vi "configuration UI.vi"() -> ()   [LabVIEW 2014, in "io editor node.lvclass"]
uses:
  io editor node.lvclass
  <vilib>/NI/Module Execution Interface/Engine Configuration/engine configuration.lvclass
  <vilib>/NI/DCAF/Modules/UI/configuration/UI Reference configuration.lvclass
  <vilib>/NI/Configuration Framework/Controls/EventCluster.ctl
  <vilib>/NI/Configuration Framework/NISE_CEF_TreeControl.lvlib
  <vilib>/NI/Tag Bus/tag/tag descriptor.lvclass
  <vilib>/NI/Tag Bus/tag/Data Type.ctl
  <vilib>/NI/DCAF/Tag Editor Core/Configuration Editor/Classes/Module editor node/module editor node.lvclass
  <vilib>/NI/DCAF/Tag Editor Core/Configuration Editor/Classes/Engine Parent/Engine Parent Editor Node.lvclass
  configuration/io configuration.lvclass
  <vilib>/NI/Tools/Keyed Array/KeyedArray.ctl
  <vilib>/NI/Tools/Keyed Array/Tools_KeyedArray.lvlib
  <vilib>/NI/AMC/Message.ctl
  <vilib>/NI/AMC/AMC.lvlib
  <vilib>/NI/AMC/Message Queue.ctl
  <vilib>/NI/Configuration Framework/Node/NISE_CEF_Node.lvclass
  <vilib>/NI/Configuration Framework/Node/NodeRef.ctl
  <vilib>/NI/Configuration Framework/Node/UserEventRef.ctl
panel:
  in  "Gen from VI":bool
  in  "Browse VI":bool
  out "VI":string
  in  "Tab Control":enum32{"Static Configuration"}(tab)
  in  "Bitfile exe dir":path caption="Directory"
  in  "Load FPGA":bool=TRUE
  in  "Resource":string
  in  "Gen from Bitfile":bool
  in  "Browse Bitfile":bool
  out "Bitfile":string
  in  "hidden_remove":bool
  in  "hidden_settings":bool
  in  "hidden_Add":bool
  in  "Remove Button":bool
  in  "Add Button":bool
  in  "channel":i32(listbox)
  in  "settings":bool
  in  "user event":T1
  in  "main queue":T2
  in  "node ref":T3
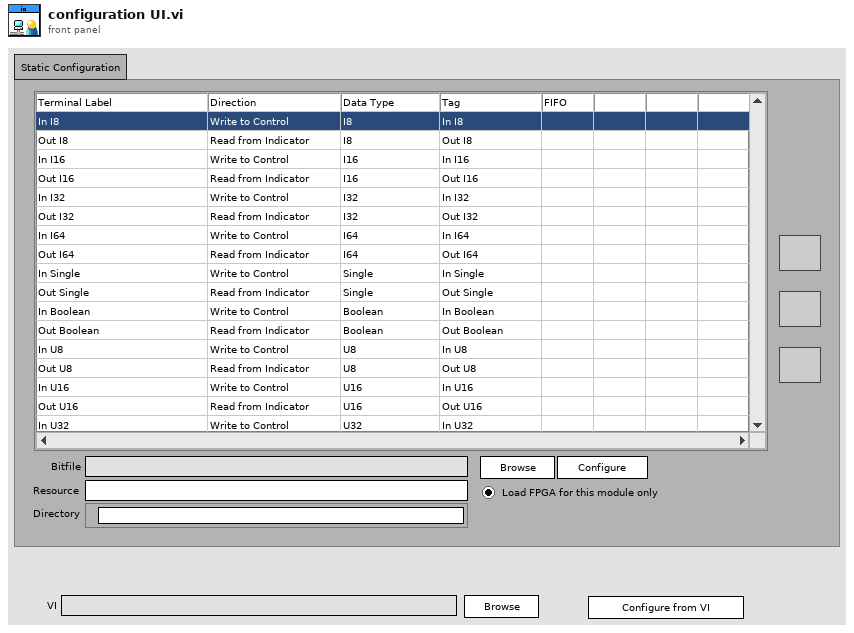
[diagram p1: front panel]
types:
  T1 = typedef "NISE_CEF_Node.lvclass/UserEventRef.ctl" = refnum<user-event>
  T2 = typedef "AMC.lvlib/Message Queue.ctl" = refnum<queue>
  T3 = typedef "NISE_CEF_Node.lvclass/NodeRef.ctl" = refnum<data-value>
  T4 = typedef "NISE_CEF_TreeControl.lvlib/EventCluster.ctl" = cluster{"command":string, "data":string}
  T5 = typedef "tag bus.lvlib/tag descriptor.lvclass/Data Type.ctl" = enum16{"Double", "Single", "I64", "I32", "I16", "I8", "U64", "U32", "U16", "U8", "Boolean", "String", "Array of Double", "Array of Single", "Array of I64", "Array of I32", "Array of I16", "Array of I8", "Array of U64", "Array of U32", "Array of U16", "Array of U8", "Array of Boolean", "Array of String"}
  T6 = typedef "io editor node.lvclass/table line.ctl" = cluster{"channel":refnum<class "TBM channel.lvclass">, "tag name":string}
  T7 = typedef "LVPoint32TypeDef.ctl" = cluster{"Horizontal":i32, "Vertical":i32}
  T8 = typedef "LVRowAndColumnTypeDef.ctl" = cluster{"Row":i32, "Column":i32}
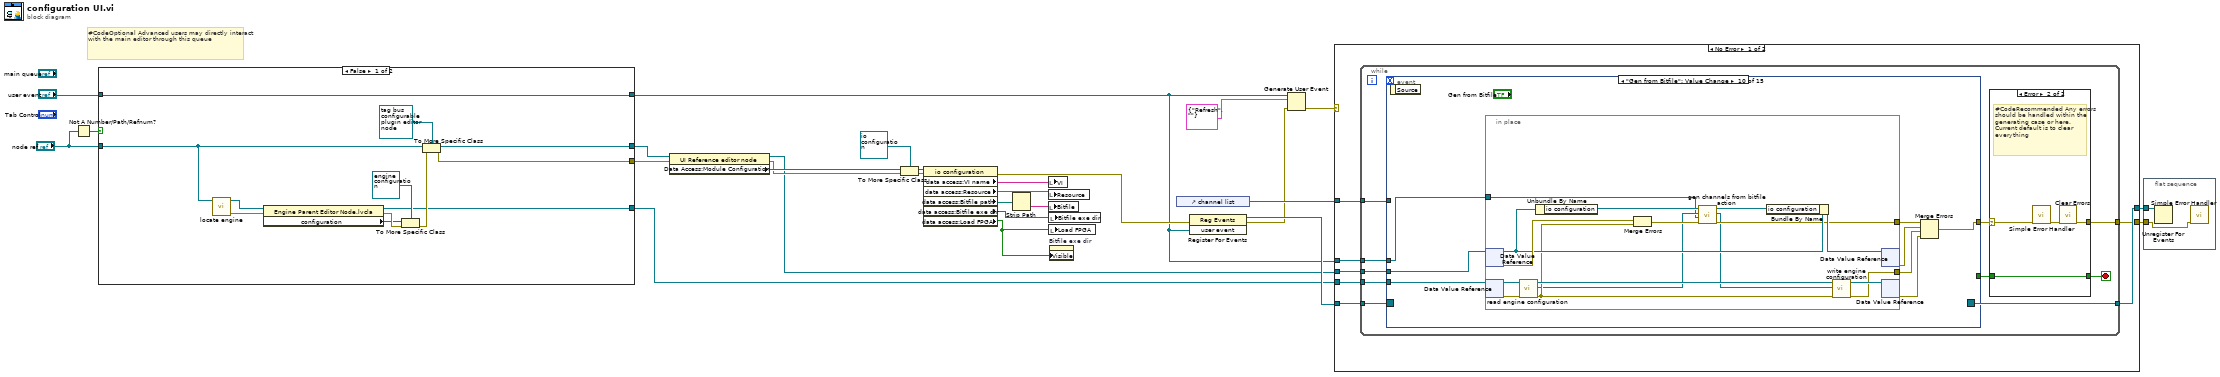
[diagram p0: block diagram]
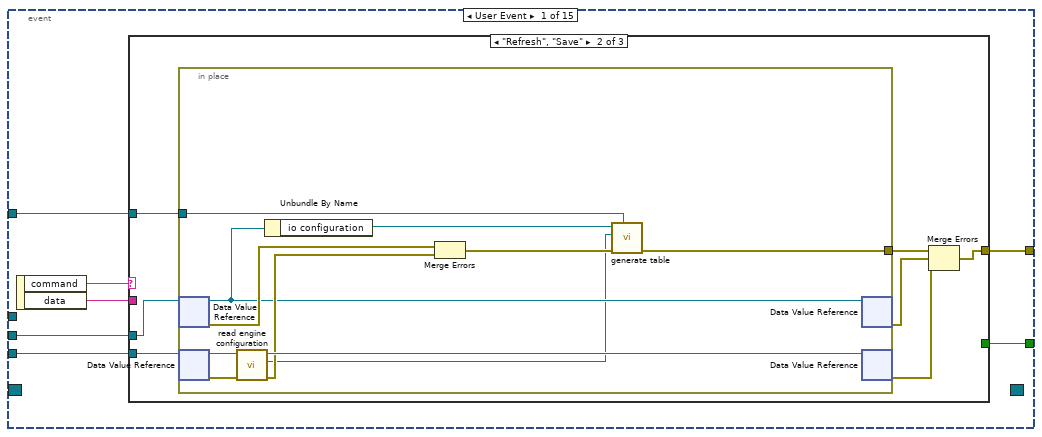
[diagram p3: hidden frame]
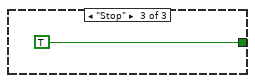
[diagram p5: hidden frame]
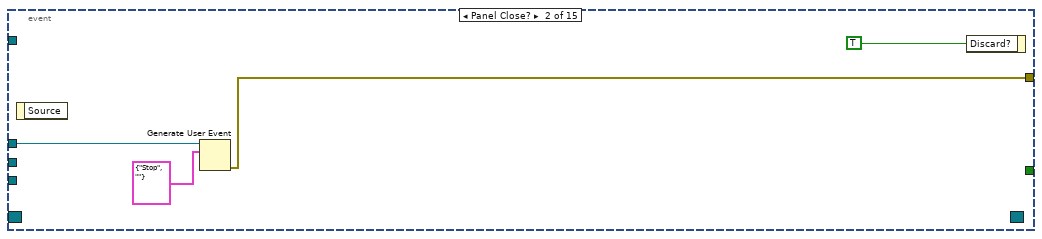
[diagram p6: hidden frame]
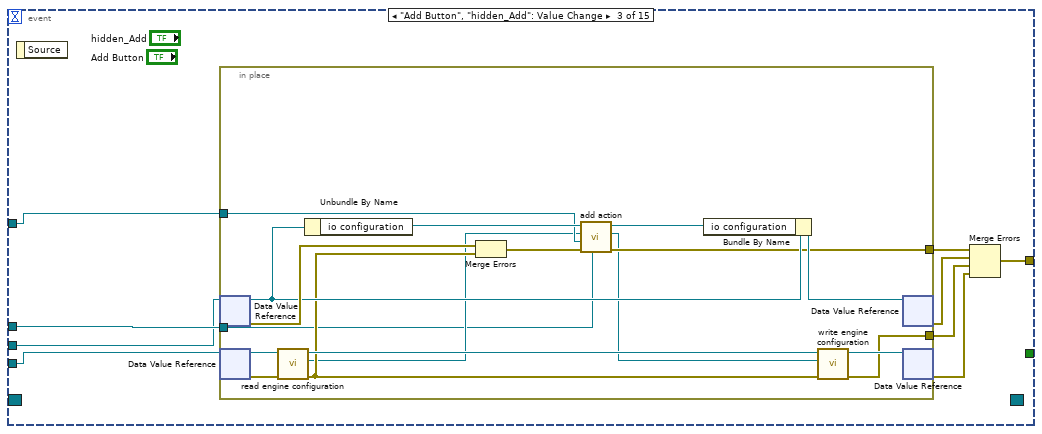
[diagram p7: hidden frame]
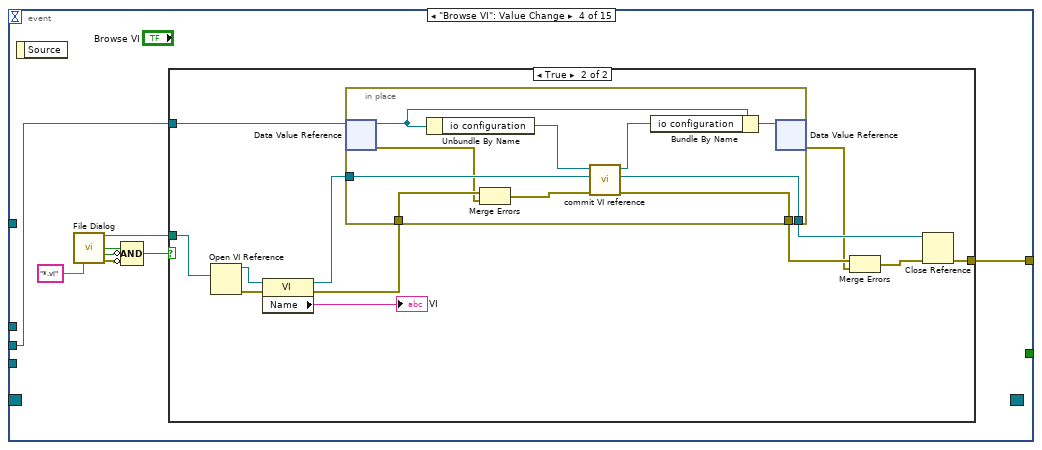
[diagram p8: hidden frame]
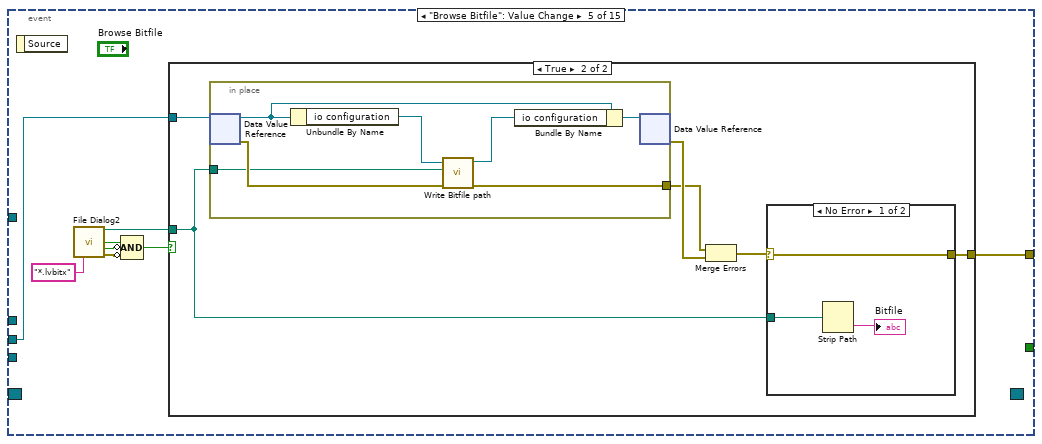
[diagram p10: hidden frame]
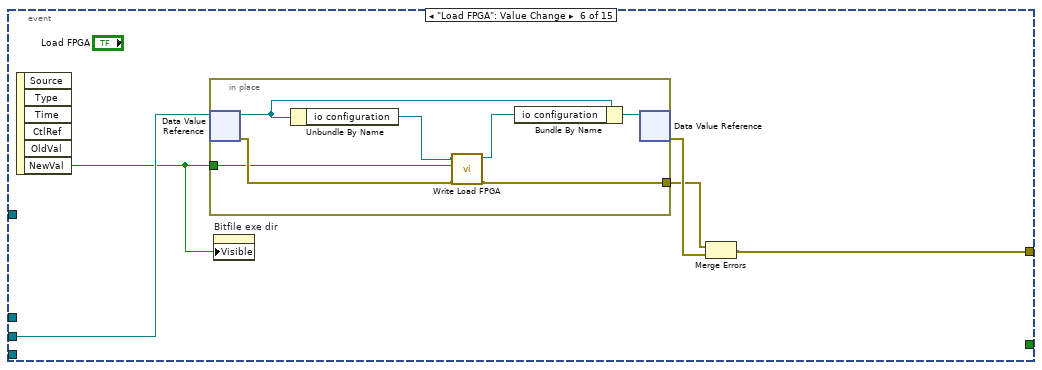
[diagram p13: hidden frame]
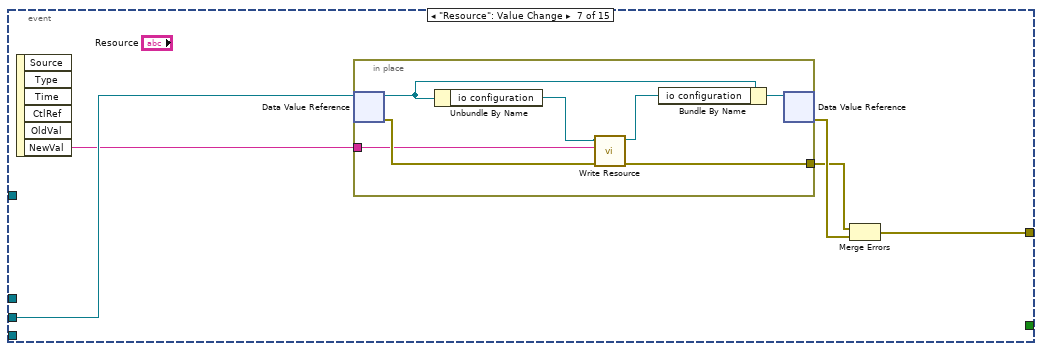
[diagram p14: hidden frame]
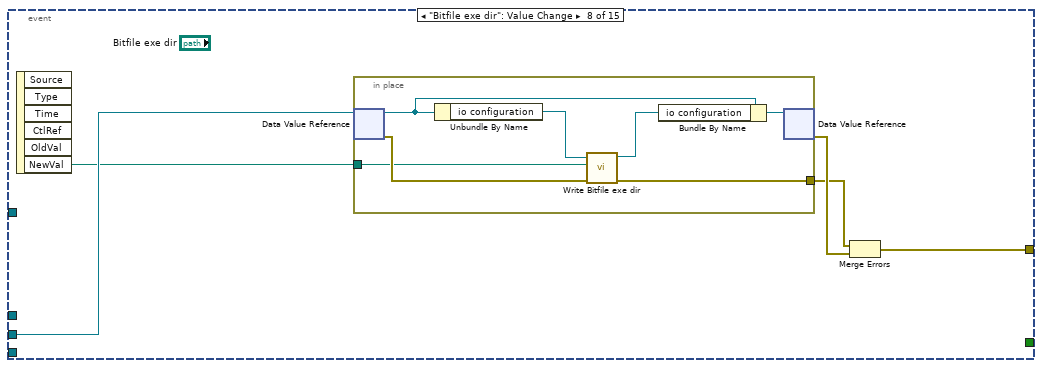
[diagram p15: hidden frame]
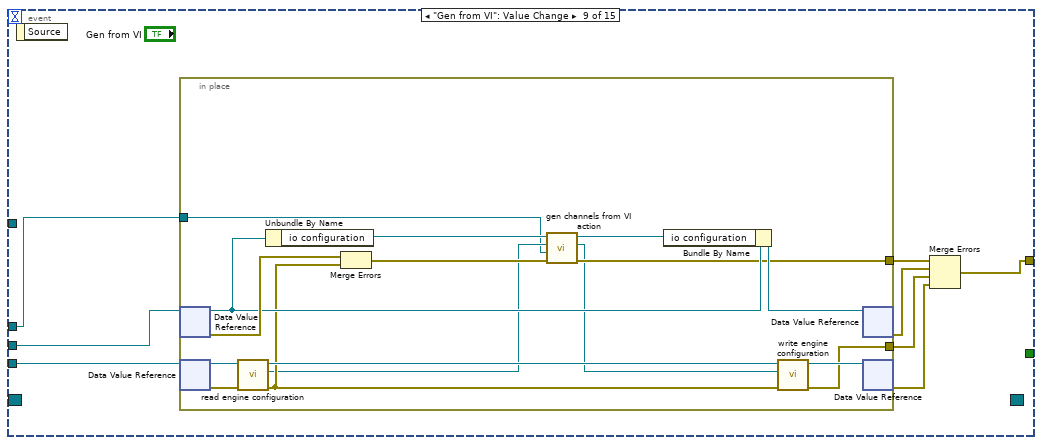
[diagram p16: hidden frame]
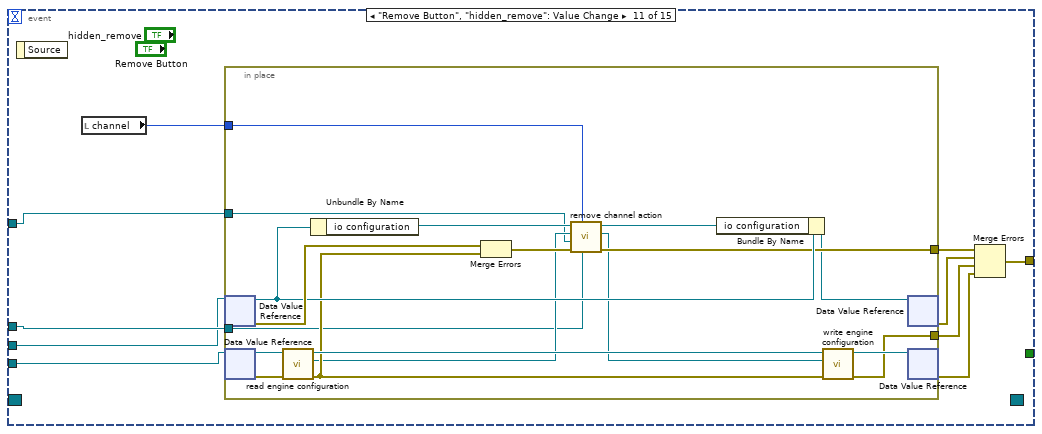
[diagram p17: hidden frame]
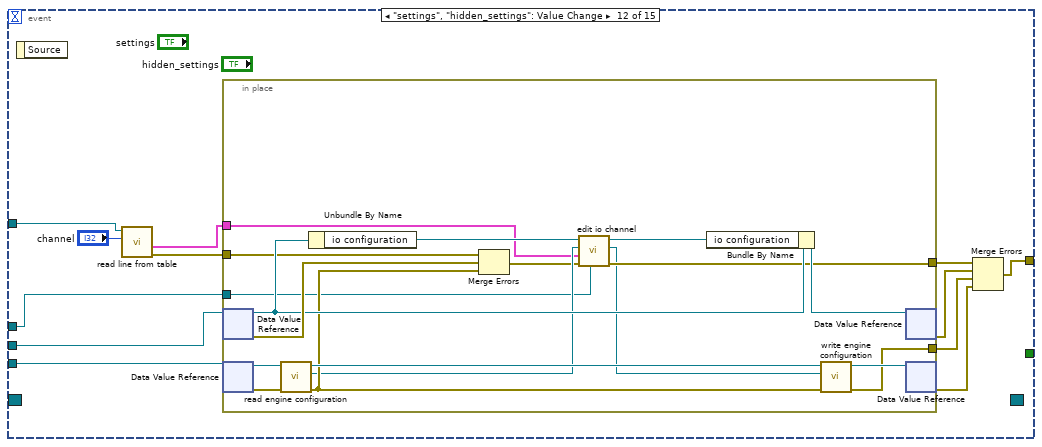
[diagram p18: hidden frame]
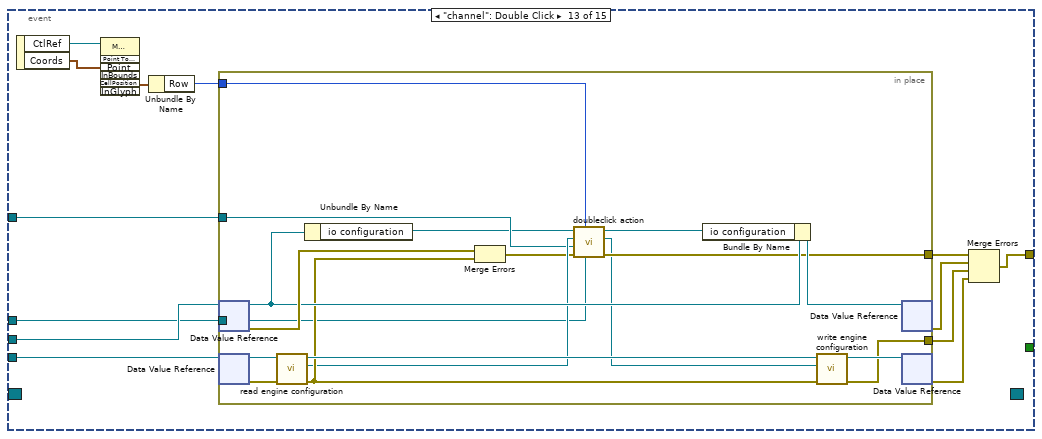
[diagram p19: hidden frame]
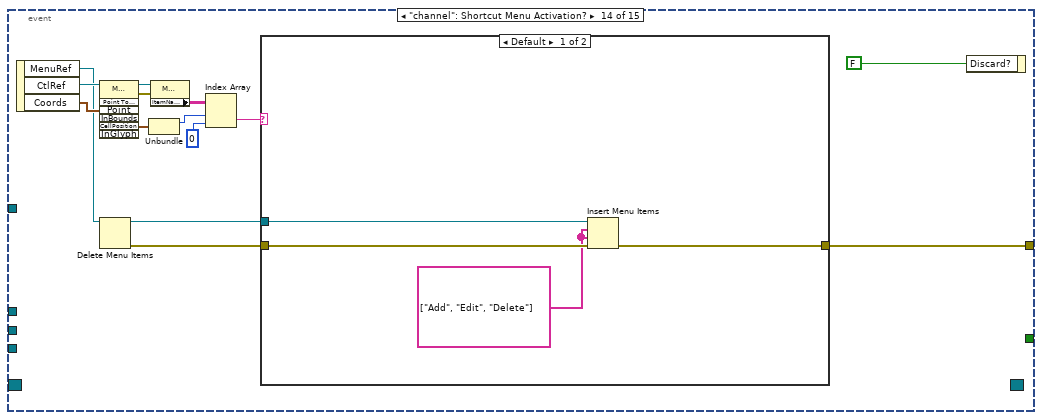
[diagram p20: hidden frame]
diagram:
  # "#CodeOptional Advanced users may directly interact with the main editor through this queue"
  n1 = Not A Number/Path/Refnum?(number/path/refnum="node ref") -> (NaN/Path/Refnum?=w21:bool)
  n2 = case shown="False" w21 {
    tunnel: "user event" -> [w39 w45]
    tunnel: [w39 w46] -> w9
    tunnel: "node ref" -> [w37 _]
    tunnel: [w36 w61] -> w16
    tunnel: [w35 w43] -> w19
    tunnel: [w28 w41] -> w14
    frame False {
      n3 = call <vilib>:"locate engine.vi"("component"=w37) -> ("error out"=w32:errorcluster, "engine"=w34:refnum<data-value>)  [unwired: 9 in]
      n4 = property class="Engine Parent Editor Node.lvcla"(reference=w34, error in=w32) -> (reference out=w28:refnum<data-value>, error out=w31:errorcluster, "configuration"=w30:refnum<class "NISE_CEF_serializable configuration.lvclass">)
      n5 = To More Specific Class(target class=refnum<class "engine configuration.lvclass"> refnum ("engine configuration.lvclass"), reference=w30, error in=w31) -> (error out=w29:errorcluster)  [unwired: 1 out]
      n6 = To More Specific Class(target class=refnum<data-value> refnum ("data value reference"), reference=w37, error in=w29) -> (specific class reference=w36:refnum<data-value>, error out=w35:errorcluster)
    }
    frame True {
      n7 = New Data Value Reference(data value=refnum<class "io editor node.lvclass"> refnum ("tag bus configurable plugin editor node")) -> (data value reference=w60:refnum<data-value>, error out=w63:errorcluster)  [unwired: 1 in]
      n8 = call-dynamic "Initialize.vi"("Engine in"=refnum<class "Engine Parent Editor Node.lvclass"> refnum) -> ("data value reference"=w59:T3)  [unwired: 8 in, 2 out]
      n9 = Create User Event(user event datatype=T4 {"command"="", "data"=""} ("event data"), error in=w63) -> (user event=w66:refnum<user-event>, error out=w62:errorcluster)
      n10 = property class="tag descriptor"(reference=refnum<class "tag descriptor.lvclass"> refnum ("tag descriptor"), "accessors:name"="mydouble" ("name"), "accessors:data type"=Data_Type."Double" ("data type")) -> (reference out=w47:refnum<class "tag descriptor.lvclass">)  [unwired: 1 in, 1 out]
      n11 = To More Specific Class(target class=refnum<data-value> refnum ("data value reference"), reference=w59) -> (specific class reference=w42:refnum<data-value>)  [unwired: 1 in, 1 out]
      n12 = property class="UI Reference editor node"(reference=w60, error in=w62, "configuration"=refnum<class "UI Reference configuration.lvclass"> refnum ("tag bus configurable plugin module configuration")) -> (reference out=w61:refnum<data-value>, error out=w53:errorcluster)
      n13 = property class="tag descriptor"(reference=w47, "accessors:name"="mydouble2" ("name")) -> (reference out=w48:refnum<class "tag descriptor.lvclass">)  [unwired: 1 in, 1 out]
      n14 = Type Cast(type=w45, x=w66) -> (*(type *) &x=w46:T1)
      n15 = call-dynamic "add tag.vi"("error in"=w53, "tag descriptor"=w47, "engine configuration in"=refnum<class "engine configuration.lvclass"> refnum ("Engine Configuration")) -> ("error out"=w51:errorcluster, "engine configuration out"=w50:refnum<class "engine configuration.lvclass">)  [unwired: 7 in]
      n16 = call-dynamic "add tag.vi"("error in"=w51, "tag descriptor"=w48, "engine configuration in"=w50) -> ("error out"=w49:errorcluster, "engine configuration out"=w40:refnum<class "engine configuration.lvclass">)  [unwired: 7 in]
      n17 = property class="Engine Parent Editor Node.lvcla"(reference=w42, error in=w49, "Data Access:Engine Configuration"=w40) -> (reference out=w41:refnum<data-value>, error out=w43:errorcluster)
    }
  }
  n18 = property class="UI Reference editor node"(reference=w16, error in=w19) -> (reference out=w15:refnum<data-value>, error out=w22:errorcluster, "Data Access:Module Configuration"=w23:refnum<class "TBM module configuration.lvclass">)
  n19 = To More Specific Class(target class=refnum<class "io configuration.lvclass"> refnum ("tag bus configurable plugin module configuration"), reference=w23, error in=w22) -> (specific class reference=w11:refnum<class "io configuration.lvclass">, error out=w17:errorcluster)
  n20 = property class="io configuration"(reference=w11, error in=w17) -> (error out=w12:errorcluster, "data access:VI name"=w10:string, "data access:Resource"=w4:string, "data access:Bitfile path"=w5:path, "data access:Bitfile exe dir"=w2:path, "data access:Load FPGA"=w1:bool)  [unwired: 1 out]
  n21 = Strip Path(path=w5) -> (name=w3:string)  [unwired: 1 out]
  n22 = local write "VI"(w10) -> ()
  n23 = local write "Resource"(w4) -> ()
  n24 = local write "Bitfile"(w3) -> ()
  n25 = local write "Bitfile exe dir"(w2) -> ()
  n26 = local write "Load FPGA"(w1) -> ()
  n27 = property on="Bitfile exe dir" class="Path"("Visible"=w1) -> ()  [unwired: 2 in, 2 out]
  n28 = control-ref of="channel list"() -> (w13:refnum<vi>)
  n29 = register-events(error in=w12, w9) -> (reference out=w27:refnum<event-registration>, error out=w7:errorcluster)  [unwired: 1 in]
  n30 = Generate User Event(user event=w9, event data cluster=T4 {"command"="Refresh", "data"=""} ("event data"), error in=w7) -> (error out=w6:errorcluster)  [unwired: 1 in, 1 out]
  n31 = case shown="No Error" w6 {
    selector: w6 -> [_ w414]
    tunnel: w27 -> [w74 w415]
    tunnel: [w73 w415] -> w26
    tunnel: [w72 w414] -> w25
    tunnel: w15 -> [w71 _]
    tunnel: w14 -> [w70 _]
    tunnel: w13 -> [w69 _]
    tunnel: w9 -> [w68 _]
    frame No Error {
      n32 = while {
        tunnel: w74 -> [w84]
        tunnel: [w83] -> w73
        tunnel: w71 -> [w79]
        tunnel: w70 -> [w78]
        tunnel: w68 -> [w77]
        tunnel: w69 -> [w75]
        tunnel: [w80] -> w72
        stop <- w82 stop-if-true
        n33 = event shown="[9] \"Gen from Bitfile\": Value Change" {
          selector: w84 -> [_ _ _ _ _ _ _ _ _ _ _ _ _ _ _]
          dyn-events: [_ _ _ _ _ _ _ _ _ _ _ _ _ _ _] -> w83
          timeout: _ -> [_ _ _ _ _ _ _ _ _ _ _ _ _ _ _]
          tunnel: [w97 _ _ _ _ _ _ _ _ _ _ _ _ _ _] -> w81
          tunnel: [w92 w117 w125 w148 w177 w203 w217 w229 w241 w265 w291 w319 w349 w375 w400] -> w76
          tunnel: w79 -> [w95 _ w121 w147 w178 w206 w218 w230 w239 w263 w286 w317 w347 _ _]
          tunnel: w78 -> [w94 _ w124 _ _ _ _ _ w240 w264 w287 w318 w348 _ _]
          tunnel: w77 -> [_ w118 w122 _ _ _ _ _ w238 w262 w289 w315 w346 _ _]
          tunnel: w75 -> [w91 _ w123 _ _ _ _ _ _ _ w288 w324 w345 _ _]
          event User Event {
            n34 = event-data() -> ("command"=w96:string, "data"=w93:string)  [unwired: 1 in]
            n35 = case shown="\"Refresh\", \"Save\"" w96 {
              tunnel: [_ _ TRUE] -> w97
              tunnel: w95 -> [_ w100 _]
              tunnel: w94 -> [_ w101 _]
              tunnel: w93 -> [_ _ _]
              tunnel: [_ w102 _] -> w92
              tunnel: w91 -> [_ w103 _]
              frame Default {
              }
              frame "Refresh", "Save" {
                n36 = in-place {
                  in-place-border: [w115] -> w104
                  in-place-border: w103 -> [w114]
                  n37 = in-place-dvr #1(w100) -> (w107:refnum<class "io editor node.lvclass">, w108:errorcluster)
                  n38 = in-place-dvr #2(w101) -> (w112:refnum<class "Engine Parent Editor Node.lvclass">, w111:errorcluster)
                  n39 = call <vilib>:"read engine configuration.vi"("error in"=w111, "Engine Parent Editor Node in"=w112) -> ("error out"=w109:errorcluster, "engine configuration"=w105:refnum<class "engine configuration.lvclass">, "Engine Parent Editor Node out"=w110:refnum<class "Engine Parent Editor Node.lvclass">)  [unwired: 7 in]
                  n40 = Unbundle By Name(w107) -> ("io configuration"=w106:refnum<class "io configuration.lvclass">)
                  n41 = Merge Errors(w108, w109) -> (w113:errorcluster)
                  n42 = call "generate table.vi"("table"=w114, "error in"=w113, "engine configuration"=w105, "tag bus configurable plugin module configuration"=w106) -> ("error out"=w115:errorcluster)  [unwired: 7 in]
                  n43 = in-place-dvr #1(w107) -> (w98:errorcluster)  [unwired: 1 out]
                  n44 = in-place-dvr #2(w110) -> (w99:errorcluster)  [unwired: 1 out]
                }
                n45 = Merge Errors(w104, w98, w99) -> (w102:errorcluster)
              }
              frame "Stop" {
              }
            }
          }
          event Panel Close? {
            n46 = event-data() -> ()  [unwired: 1 in, 1 out]
            n47 = Generate User Event(user event=w118, event data cluster=T4 {"command"="Stop", "data"=""} ("event data")) -> (error out=w117:errorcluster)  [unwired: 2 in, 1 out]
            n48 = event-data("Discard?"=TRUE) -> ()  [unwired: 1 in, 1 out]
          }
          event "Add Button", "hidden_Add": Value Change {
            n49 = event-data() -> ()  [unwired: 1 in, 1 out]
            n50 = in-place {
              in-place-border: [w137] -> w126
              in-place-border: [w140] -> w129
              in-place-border: w123 -> [w132]
              in-place-border: w122 -> [w130]
              n51 = in-place-dvr #3(w121) -> (w143:refnum<class "io editor node.lvclass">, w144:errorcluster)
              n52 = in-place-dvr #4(w124) -> (w146:refnum<class "Engine Parent Editor Node.lvclass">, w145:errorcluster)
              n53 = call <vilib>:"read engine configuration.vi"("error in"=w145, "Engine Parent Editor Node in"=w146) -> ("error out"=w139:errorcluster, "engine configuration"=w131:refnum<class "engine configuration.lvclass">, "Engine Parent Editor Node out"=w142:refnum<class "Engine Parent Editor Node.lvclass">)  [unwired: 7 in]
              n54 = Unbundle By Name(w143) -> ("io configuration"=w133:refnum<class "io configuration.lvclass">)
              n55 = Merge Errors(w144, w139) -> (w136:errorcluster)
              n56 = call "add action.vi"("user event"=w130, "error in"=w136, "channel list"=w132, "engine configuration in"=w131, "io configuration in"=w133) -> ("error out"=w137:errorcluster, "engine configuration out"=w134:refnum<class "engine configuration.lvclass">, "io configuration out"=w135:refnum<class "io configuration.lvclass">)  [unwired: 4 in]
              n57 = Bundle By Name(cluster=w143, "io configuration"=w135) -> (w138:refnum<class "io editor node.lvclass">)
              n58 = call <vilib>:"write engine configuration.vi"("error in"=w139, "engine configuration"=w134, "Engine Parent Editor Node in"=w142) -> ("error out"=w140:errorcluster, "Engine Parent Editor Node out"=w141:refnum<class "Engine Parent Editor Node.lvclass">)  [unwired: 7 in]
              n59 = in-place-dvr #3(w138) -> (w128:errorcluster)  [unwired: 1 out]
              n60 = in-place-dvr #4(w141) -> (w127:errorcluster)  [unwired: 1 out]
            }
            n61 = Merge Errors(w126, w128, w129, w127) -> (w125:errorcluster)
          }
          event "Browse VI": Value Change {
            n62 = event-data() -> ()  [unwired: 1 in, 1 out]
            n63 = call "File Dialog"("pattern (all files)"="*.vi") -> ("selected path"=w149:path, "exists"=w153:bool, "cancelled"=w152:bool, "error out"=w151:errorcluster)  [unwired: 11 in]
            n64 = Compound Arithmetic op=AND(w153, invert w152, invert w151) -> (w150:bool)
            n65 = case shown="True" w150 {
              tunnel: w149 -> [_ w166]
              tunnel: [_ w162] -> w148
              tunnel: w147 -> [_ w157]
              frame False {
              }
              frame True {
                n66 = Open VI Reference(vi path=w166) -> (vi reference=w164:refnum<vi>, error out=w165:errorcluster)  [unwired: 5 in]
                n67 = property class="VI"(reference=w164, error in=w165) -> (reference out=w159:refnum<vi>, error out=w160:errorcluster, "Name"=→"VI":string)
                n68 = in-place {
                  in-place-border: [w176] -> w161
                  in-place-border: w160 -> [w175]
                  in-place-border: w159 -> [w174]
                  in-place-border: [w173] -> w158
                  n69 = in-place-dvr #5(w157) -> (w170:refnum<class "io editor node.lvclass">, w167:errorcluster)
                  n70 = Unbundle By Name(w170) -> ("io configuration"=w172:refnum<class "io configuration.lvclass">)
                  n71 = Merge Errors(w175, w167) -> (w168:errorcluster)
                  n72 = call "commit VI reference.vi"("error in"=w168, "VI Refnum in"=w174, "io configuration in"=w172) -> ("error out"=w173:errorcluster, "VI Refnum out"=w176:refnum<vi>, "io configuration out"=w169:refnum<class "io configuration.lvclass">)  [unwired: 6 in]
                  n73 = Bundle By Name(cluster=w170, "io configuration"=w169) -> (w171:refnum<class "io editor node.lvclass">)
                  n74 = in-place-dvr #5(w171) -> (w155:errorcluster)  [unwired: 1 out]
                }
                n75 = Merge Errors(w158, w155) -> (w156:errorcluster)
                n76 = Close Reference(reference=w161, error in (no error)=w156) -> (error out=w162:errorcluster)
              }
            }
          }
          event "Browse Bitfile": Value Change {
            n77 = event-data() -> ()  [unwired: 1 in, 1 out]
            n78 = call "File Dialog2"("pattern (all files)"="*.lvbitx") -> ("selected path"=w179:path, "exists"=w183:bool, "cancelled"=w182:bool, "error out"=w181:errorcluster)  [unwired: 11 in]
            n79 = Compound Arithmetic op=AND(w183, invert w182, invert w181) -> (w180:bool)
            n80 = case shown="True" w180 {
              tunnel: w179 -> [_ w186]
              tunnel: w178 -> [_ w190]
              tunnel: [_ w185] -> w177
              frame False {
              }
              frame True {
                n81 = in-place {
                  in-place-border: [w196] -> w188
                  in-place-border: w186 -> [w195]
                  n82 = in-place-dvr #6(w190) -> (w200:refnum<class "io editor node.lvclass">, w197:errorcluster)
                  n83 = Unbundle By Name(w200) -> ("io configuration"=w199:refnum<class "io configuration.lvclass">)
                  n84 = call "Write Bitfile path.vi"("error in (no error)"=w197, "Bitfile path"=w195, "io configuration in"=w199) -> ("error out"=w196:errorcluster, "io configuration out"=w198:refnum<class "io configuration.lvclass">)  [unwired: 7 in]
                  n85 = Bundle By Name(cluster=w200, "io configuration"=w198) -> (w201:refnum<class "io editor node.lvclass">)
                  n86 = in-place-dvr #6(w201) -> (w189:errorcluster)  [unwired: 1 out]
                }
                n87 = Merge Errors(w188, w189) -> (w187:errorcluster)
                n88 = case shown="No Error" w187 {
                  selector: w187 -> [w191 w194]
                  tunnel: w186 -> [w192 _]
                  tunnel: [w191 w194] -> w185
                  frame No Error {
                    n89 = Strip Path(path=w192) -> (name=→"Bitfile":string)  [unwired: 1 out]
                  }
                  frame Error {
                  }
                }
              }
            }
          }
          event "Load FPGA": Value Change {
            n90 = event-data() -> ("NewVal"=w202:bool)  [unwired: 1 in, 5 out]
            n91 = in-place {
              in-place-border: [w208] -> w204
              in-place-border: w202 -> [w207]
              n92 = in-place-dvr #7(w206) -> (w212:refnum<class "io editor node.lvclass">, w209:errorcluster)
              n93 = Unbundle By Name(w212) -> ("io configuration"=w211:refnum<class "io configuration.lvclass">)
              n94 = call "Write Load FPGA.vi"("error in (no error)"=w209, "Load FPGA"=w207, "io configuration in"=w211) -> ("error out"=w208:errorcluster, "io configuration out"=w210:refnum<class "io configuration.lvclass">)  [unwired: 7 in]
              n95 = Bundle By Name(cluster=w212, "io configuration"=w210) -> (w213:refnum<class "io editor node.lvclass">)
              n96 = in-place-dvr #7(w213) -> (w205:errorcluster)  [unwired: 1 out]
            }
            n97 = property on="Bitfile exe dir" class="Path"("Visible"=w202) -> ()  [unwired: 2 in, 2 out]
            n98 = Merge Errors(w204, w205) -> (w203:errorcluster)
          }
          event "Resource": Value Change {
            n99 = event-data() -> ("NewVal"=w214:string)  [unwired: 1 in, 5 out]
            n100 = in-place {
              in-place-border: [w220] -> w215
              in-place-border: w214 -> [w219]
              n101 = in-place-dvr #8(w218) -> (w224:refnum<class "io editor node.lvclass">, w221:errorcluster)
              n102 = Unbundle By Name(w224) -> ("io configuration"=w223:refnum<class "io configuration.lvclass">)
              n103 = call "Write Resource.vi"("error in (no error)"=w221, "Resource"=w219, "io configuration in"=w223) -> ("error out"=w220:errorcluster, "io configuration out"=w222:refnum<class "io configuration.lvclass">)  [unwired: 7 in]
              n104 = Bundle By Name(cluster=w224, "io configuration"=w222) -> (w225:refnum<class "io editor node.lvclass">)
              n105 = in-place-dvr #8(w225) -> (w216:errorcluster)  [unwired: 1 out]
            }
            n106 = Merge Errors(w215, w216) -> (w217:errorcluster)
          }
          event "Bitfile exe dir": Value Change {
            n107 = event-data() -> ("NewVal"=w226:path)  [unwired: 1 in, 5 out]
            n108 = in-place {
              in-place-border: [w232] -> w227
              in-place-border: w226 -> [w231]
              n109 = in-place-dvr #9(w230) -> (w236:refnum<class "io editor node.lvclass">, w233:errorcluster)
              n110 = Unbundle By Name(w236) -> ("io configuration"=w235:refnum<class "io configuration.lvclass">)
              n111 = call "Write Bitfile exe dir.vi"("error in (no error)"=w233, "Bitfile exe dir"=w231, "io configuration in"=w235) -> ("error out"=w232:errorcluster, "io configuration out"=w234:refnum<class "io configuration.lvclass">)  [unwired: 7 in]
              n112 = Bundle By Name(cluster=w236, "io configuration"=w234) -> (w237:refnum<class "io editor node.lvclass">)
              n113 = in-place-dvr #9(w237) -> (w228:errorcluster)  [unwired: 1 out]
            }
            n114 = Merge Errors(w227, w228) -> (w229:errorcluster)
          }
          event "Gen from VI": Value Change {
            n115 = event-data() -> ()  [unwired: 1 in, 1 out]
            n116 = in-place {
              in-place-border: [w252] -> w242
              in-place-border: [w255] -> w245
              in-place-border: w238 -> [w246]
              n117 = in-place-dvr #10(w239) -> (w258:refnum<class "io editor node.lvclass">, w259:errorcluster)
              n118 = in-place-dvr #11(w240) -> (w261:refnum<class "Engine Parent Editor Node.lvclass">, w260:errorcluster)
              n119 = call <vilib>:"read engine configuration.vi"("error in"=w260, "Engine Parent Editor Node in"=w261) -> ("error out"=w254:errorcluster, "engine configuration"=w250:refnum<class "engine configuration.lvclass">, "Engine Parent Editor Node out"=w257:refnum<class "Engine Parent Editor Node.lvclass">)  [unwired: 7 in]
              n120 = Unbundle By Name(w258) -> ("io configuration"=w249:refnum<class "io configuration.lvclass">)
              n121 = Merge Errors(w259, w254) -> (w251:errorcluster)
              n122 = call "gen channels from VI action.vi"("error in"=w251, "user event"=w246, "engine configuration in"=w250, "io configuration in"=w249) -> ("error out"=w252:errorcluster, "engine configuration out"=w247:refnum<class "engine configuration.lvclass">, "io configuration out"=w248:refnum<class "io configuration.lvclass">)  [unwired: 5 in]
              n123 = Bundle By Name(cluster=w258, "io configuration"=w248) -> (w253:refnum<class "io editor node.lvclass">)
              n124 = call <vilib>:"write engine configuration.vi"("error in"=w254, "engine configuration"=w247, "Engine Parent Editor Node in"=w257) -> ("error out"=w255:errorcluster, "Engine Parent Editor Node out"=w256:refnum<class "Engine Parent Editor Node.lvclass">)  [unwired: 7 in]
              n125 = in-place-dvr #10(w253) -> (w244:errorcluster)  [unwired: 1 out]
              n126 = in-place-dvr #11(w256) -> (w243:errorcluster)  [unwired: 1 out]
            }
            n127 = Merge Errors(w242, w244, w245, w243) -> (w241:errorcluster)
          }
          event "Gen from Bitfile": Value Change {
            n128 = event-data() -> ()  [unwired: 1 in, 1 out]
            n129 = in-place {
              in-place-border: [w276] -> w266
              in-place-border: [w279] -> w269
              in-place-border: w262 -> [w270]
              n130 = in-place-dvr #12(w263) -> (w282:refnum<class "io editor node.lvclass">, w283:errorcluster)
              n131 = in-place-dvr #13(w264) -> (w285:refnum<class "Engine Parent Editor Node.lvclass">, w284:errorcluster)
              n132 = call <vilib>:"read engine configuration.vi"("error in"=w284, "Engine Parent Editor Node in"=w285) -> ("error out"=w278:errorcluster, "engine configuration"=w274:refnum<class "engine configuration.lvclass">, "Engine Parent Editor Node out"=w281:refnum<class "Engine Parent Editor Node.lvclass">)  [unwired: 7 in]
              n133 = Unbundle By Name(w282) -> ("io configuration"=w273:refnum<class "io configuration.lvclass">)
              n134 = Merge Errors(w283, w278) -> (w275:errorcluster)
              n135 = call "gen channels from bitfile action.vi"("error in"=w275, "user event"=w270, "engine configuration in"=w274, "io configuration in"=w273) -> ("error out"=w276:errorcluster, "engine configuration out"=w271:refnum<class "engine configuration.lvclass">, "io configuration out"=w272:refnum<class "io configuration.lvclass">)  [unwired: 5 in]
              n136 = Bundle By Name(cluster=w282, "io configuration"=w272) -> (w277:refnum<class "io editor node.lvclass">)
              n137 = call <vilib>:"write engine configuration.vi"("error in"=w278, "engine configuration"=w271, "Engine Parent Editor Node in"=w281) -> ("error out"=w279:errorcluster, "Engine Parent Editor Node out"=w280:refnum<class "Engine Parent Editor Node.lvclass">)  [unwired: 7 in]
              n138 = in-place-dvr #12(w277) -> (w268:errorcluster)  [unwired: 1 out]
              n139 = in-place-dvr #13(w280) -> (w267:errorcluster)  [unwired: 1 out]
            }
            n140 = Merge Errors(w266, w268, w269, w267) -> (w265:errorcluster)
          }
          event "Remove Button", "hidden_remove": Value Change {
            n141 = event-data() -> ()  [unwired: 1 in, 1 out]
            n142 = local read "channel"() -> (w290:i32)
            n143 = in-place {
              in-place-border: [w305] -> w292
              in-place-border: [w307] -> w295
              in-place-border: w290 -> [w300]
              in-place-border: w289 -> [w299]
              in-place-border: w288 -> [w298]
              n144 = in-place-dvr #14(w286) -> (w310:refnum<class "io editor node.lvclass">, w311:errorcluster)
              n145 = in-place-dvr #15(w287) -> (w313:refnum<class "Engine Parent Editor Node.lvclass">, w312:errorcluster)
              n146 = call <vilib>:"read engine configuration.vi"("error in"=w312, "Engine Parent Editor Node in"=w313) -> ("error out"=w306:errorcluster, "engine configuration"=w303:refnum<class "engine configuration.lvclass">, "Engine Parent Editor Node out"=w309:refnum<class "Engine Parent Editor Node.lvclass">)  [unwired: 7 in]
              n147 = Unbundle By Name(w310) -> ("io configuration"=w301:refnum<class "io configuration.lvclass">)
              n148 = Merge Errors(w311, w306) -> (w304:errorcluster)
              n149 = call "remove channel action.vi"("user event"=w299, "channel"=w300, "error in"=w304, "channel list"=w298, "engine configuration in"=w303, "io configuration in"=w301) -> ("error out"=w305:errorcluster, "engine configuration out"=w302:refnum<class "engine configuration.lvclass">, "io configuration out"=w296:refnum<class "io configuration.lvclass">)  [unwired: 3 in]
              n150 = Bundle By Name(cluster=w310, "io configuration"=w296) -> (w297:refnum<class "io editor node.lvclass">)
              n151 = call <vilib>:"write engine configuration.vi"("error in"=w306, "engine configuration"=w302, "Engine Parent Editor Node in"=w309) -> ("error out"=w307:errorcluster, "Engine Parent Editor Node out"=w308:refnum<class "Engine Parent Editor Node.lvclass">)  [unwired: 7 in]
              n152 = in-place-dvr #14(w297) -> (w294:errorcluster)  [unwired: 1 out]
              n153 = in-place-dvr #15(w308) -> (w293:errorcluster)  [unwired: 1 out]
            }
            n154 = Merge Errors(w292, w294, w295, w293) -> (w291:errorcluster)
          }
          event "settings", "hidden_settings": Value Change {
            n155 = event-data() -> ()  [unwired: 1 in, 1 out]
            n156 = call "read line from table.vi"("line number"="channel", "channels table"=w324) -> ("error out"=w316:errorcluster, "line"=w314:T6)  [unwired: 6 in, 2 out]
            n157 = in-place {
              in-place-border: [w333] -> w320
              in-place-border: [w337] -> w323
              in-place-border: w316 -> [w334]
              in-place-border: w315 -> [w327]
              in-place-border: w314 -> [w326]
              n158 = in-place-dvr #16(w317) -> (w340:refnum<class "io editor node.lvclass">, w341:errorcluster)
              n159 = in-place-dvr #17(w318) -> (w343:refnum<class "Engine Parent Editor Node.lvclass">, w342:errorcluster)
              n160 = call <vilib>:"read engine configuration.vi"("error in"=w342, "Engine Parent Editor Node in"=w343) -> ("error out"=w336:errorcluster, "engine configuration"=w329:refnum<class "engine configuration.lvclass">, "Engine Parent Editor Node out"=w339:refnum<class "Engine Parent Editor Node.lvclass">)  [unwired: 7 in]
              n161 = Unbundle By Name(w340) -> ("io configuration"=w330:refnum<class "io configuration.lvclass">)
              n162 = Merge Errors(w334, w341, w336) -> (w328:errorcluster)
              n163 = call "edit io channel.vi"("user event"=w327, "error in"=w328, "line"=w326, "engine configuration in"=w329, "tag bus configurable plugin module configuration in"=w330) -> ("error out"=w333:errorcluster, "engine configuration"=w331:refnum<class "engine configuration.lvclass">, "tag bus configurable plugin module configuration out"=w332:refnum<class "io configuration.lvclass">)  [unwired: 4 in]
              n164 = Bundle By Name(cluster=w340, "io configuration"=w332) -> (w335:refnum<class "io editor node.lvclass">)
              n165 = call <vilib>:"write engine configuration.vi"("error in"=w336, "engine configuration"=w331, "Engine Parent Editor Node in"=w339) -> ("error out"=w337:errorcluster, "Engine Parent Editor Node out"=w338:refnum<class "Engine Parent Editor Node.lvclass">)  [unwired: 7 in]
              n166 = in-place-dvr #16(w335) -> (w322:errorcluster)  [unwired: 1 out]
              n167 = in-place-dvr #17(w338) -> (w321:errorcluster)  [unwired: 1 out]
            }
            n168 = Merge Errors(w320, w322, w323, w321) -> (w319:errorcluster)
          }
          event "channel": Double Click {
            n169 = event-data() -> ("CtlRef"=w356:refnum<vi>, "Coords"=w355:T7)  [unwired: 1 in]
            n170 = invoke class="MCListbox (strict)" method="Point To Row Column"(reference=w356, "Point"=w355) -> ("CellPosition"=w354:T8)  [unwired: 5 in, 6 out]
            n171 = Unbundle By Name(w354) -> ("Row"=w344:i32)
            n172 = in-place {
              in-place-border: [w365] -> w350
              in-place-border: [w368] -> w353
              in-place-border: w346 -> [w361]
              in-place-border: w345 -> [w360]
              in-place-border: w344 -> [w358]
              n173 = in-place-dvr #18(w347) -> (w371:refnum<class "io editor node.lvclass">, w372:errorcluster)
              n174 = in-place-dvr #19(w348) -> (w374:refnum<class "Engine Parent Editor Node.lvclass">, w373:errorcluster)
              n175 = call <vilib>:"read engine configuration.vi"("error in"=w373, "Engine Parent Editor Node in"=w374) -> ("error out"=w367:errorcluster, "engine configuration"=w362:refnum<class "engine configuration.lvclass">, "Engine Parent Editor Node out"=w370:refnum<class "Engine Parent Editor Node.lvclass">)  [unwired: 7 in]
              n176 = Unbundle By Name(w371) -> ("io configuration"=w359:refnum<class "io configuration.lvclass">)
              n177 = Merge Errors(w372, w367) -> (w357:errorcluster)
              n178 = call "doubleclick action.vi"("user event"=w361, "Row"=w358, "error in"=w357, "channel list"=w360, "engine configuration in"=w362, "UI Reference configuration in"=w359) -> ("error out"=w365:errorcluster, "engine configuration out"=w363:refnum<class "engine configuration.lvclass">, "UI Reference configuration out"=w364:refnum<class "io configuration.lvclass">)  [unwired: 3 in]
              n179 = Bundle By Name(cluster=w371, "io configuration"=w364) -> (w366:refnum<class "io editor node.lvclass">)
              n180 = call <vilib>:"write engine configuration.vi"("error in"=w367, "engine configuration"=w363, "Engine Parent Editor Node in"=w370) -> ("error out"=w368:errorcluster, "Engine Parent Editor Node out"=w369:refnum<class "Engine Parent Editor Node.lvclass">)  [unwired: 7 in]
              n181 = in-place-dvr #18(w366) -> (w352:errorcluster)  [unwired: 1 out]
              n182 = in-place-dvr #19(w369) -> (w351:errorcluster)  [unwired: 1 out]
            }
            n183 = Merge Errors(w350, w352, w353, w351) -> (w349:errorcluster)
          }
          event "channel": Shortcut Menu Activation? {
            n184 = event-data() -> ("MenuRef"=w385:refnum<k9>, "CtlRef"=w387:refnum<vi>, "Coords"=w386:T7)  [unwired: 1 in]
            n185 = invoke class="MCListbox (strict)" method="Point To Row Column"(reference=w387, "Point"=w386) -> (reference out=w384:refnum<vi>, error out=w383:errorcluster, "CellPosition"=w382:T8)  [unwired: 5 in, 4 out]
            n186 = Delete Menu Items(9:w385) -> (0:w376:errorcluster, 3:w377:refnum<k9>)  [unwired: 3 in]
            n187 = Unbundle(w382) -> ("Row"=w380:i32)  [unwired: 1 out]
            n188 = property class="MCListbox (strict)"(reference=w384, error in=w383) -> ("ItemNames"=w381:string[][])  [unwired: 2 out]
            n189 = Index Array(array=w381, index (row)=w380, index (col)=0 ("disabled index (col)")) -> (element=w378:string)
            n190 = case shown="Default" w378 {
              tunnel: w377 -> [w392 w396]
              tunnel: w376 -> [w391 w395]
              tunnel: [w390 w394] -> w375
              frame Default {
                w389 = string[] ["Add", "Edit", "Delete"] ("item names")
                n191 = Insert Menu Items(6:w391, 7:w389, 8:w389, 9:w392) -> (0:w390:errorcluster)  [unwired: 2 in, 2 out]
              }
              frame "" {
                w393 = string[] ["Add"] ("item names")
                n192 = Insert Menu Items(6:w395, 7:w393, 8:w393, 9:w396) -> (0:w394:errorcluster)  [unwired: 2 in, 2 out]
              }
            }
            n193 = event-data("Discard?"=FALSE) -> ()  [unwired: 1 in, 1 out]
          }
          event "channel": Shortcut Menu Selection (User) {
            n194 = event-data() -> ("ItemTag"=w401:string, "CtlRef"=w402:refnum<vi>, "Coords"=w403:T7)  [unwired: 1 in]
            n195 = invoke class="MCListbox (strict)" method="Point To Row Column"(reference=w402, "Point"=w403) -> ("CellPosition"=w398:T8)  [unwired: 5 in, 6 out]
            n196 = Unbundle By Name(w398) -> ("Row"=w397:i32)
            n197 = property on="channel" class="MCListbox (strict)"("Value"=w397) -> (error out=w399:errorcluster)  [unwired: 2 in, 1 out]
            n198 = case shown="\"Add\"" w401 {
              tunnel: w399 -> [w404 w406 w410 w413]
              tunnel: [w404 w405 w409 w412] -> w400
              frame Default {
              }
              frame "Add" {
                n199 = property on="hidden_Add" class="Bool (strict)"(error in=w406, "Val(Sgnl)"=TRUE ("Value (Signaling)")) -> (error out=w405:errorcluster)  [unwired: 1 in, 1 out]
              }
              frame "Edit" {
                n200 = property on="hidden_settings" class="Bool (strict)"(error in=w410, "Val(Sgnl)"=TRUE ("Value (Signaling)")) -> (error out=w409:errorcluster)  [unwired: 1 in, 1 out]
              }
              frame "Delete" {
                n201 = property on="hidden_remove" class="Bool (strict)"(error in=w413, "Val(Sgnl)"=FALSE ("Value (Signaling)")) -> (error out=w412:errorcluster)  [unwired: 1 in, 1 out]
              }
            }
          }
        }
        n202 = case shown="Error" w76 {
          selector: w76 -> [w85 w89]
          tunnel: [w86 w90] -> w82
          tunnel: w81 -> [w86 w90]
          tunnel: [w85 w87] -> w80
          frame No Error {
          }
          frame Error {
            # "#CodeRecommended Any errors should be handled within the generating case or here. Current default is to clear everything"
            n203 = call <vilib>:"Simple Error Handler.vi"("error in (no error)"=w89) -> ("error out"=w88:errorcluster)  [unwired: 4 in, 4 out]
            n204 = call <vilib>:"Clear Errors.vi"("error in (no error)"=w88) -> ("error out"=w87:errorcluster)  [unwired: 5 in, 1 out]
          }
        }
      }
    }
    frame Error {
    }
  }
  n205 = flat-sequence {
    tunnel: w26 -> [w417]
    tunnel: w25 -> [w416]
    frame #0 {
      n206 = Unregister For Events(event registration refnum=w417) -> ()  [unwired: 1 in, 1 out]
      n207 = call <vilib>:"Simple Error Handler.vi"("error in (no error)"=w416) -> ()  [unwired: 4 in, 5 out]
    }
  }
